vi "InitializeComms.vi"(4 "Inert MFC Channel":i32=8, 6 "Active MFC Channel":i32=7, 7 "Probe Target State":T1 {"Tset" format="%.1f"; "Telem" format="%.1f"; "GasC" format="%.1g"; "GasB" format="%.1f"; "GasA" format="%.1f"; "Z" format="%.3g"; "Y" format="%.3g"; "X" format="%.3g"; "RampRate" format="%.1f"}, 8 "error in":errorcluster, 9 "MFC channel":refnum<visa-resource-name>="COM2", 10 "Watlow channel":refnum<visa-resource-name>="COM3", 11 "Motor channel":refnum<visa-resource-name>="COM6") -> (0 "error out":errorcluster, 2 "Current probe state":T1 {"Tset" format="%.1f"; "Telem" format="%.1f"; "GasC" format="%.1g"; "GasB" format="%.1f"; "GasA" format="%.1f"; "Z" format="%.3g"; "Y" format="%.3g"; "X" format="%.3g"; "RampRate" format="%.1f"}, 3 "Probe Target State out":T1 {"Tset" format="%.1f"; "Telem" format="%.1f"; "GasC" format="%.1g"; "GasB" format="%.1f"; "GasA" format="%.1f"; "Z" format="%.3g"; "Y" format="%.3g"; "X" format="%.3g"; "RampRate" format="%.1f"})   [LabVIEW 2013]
uses:
  controls/Microprobe Vars.ctl
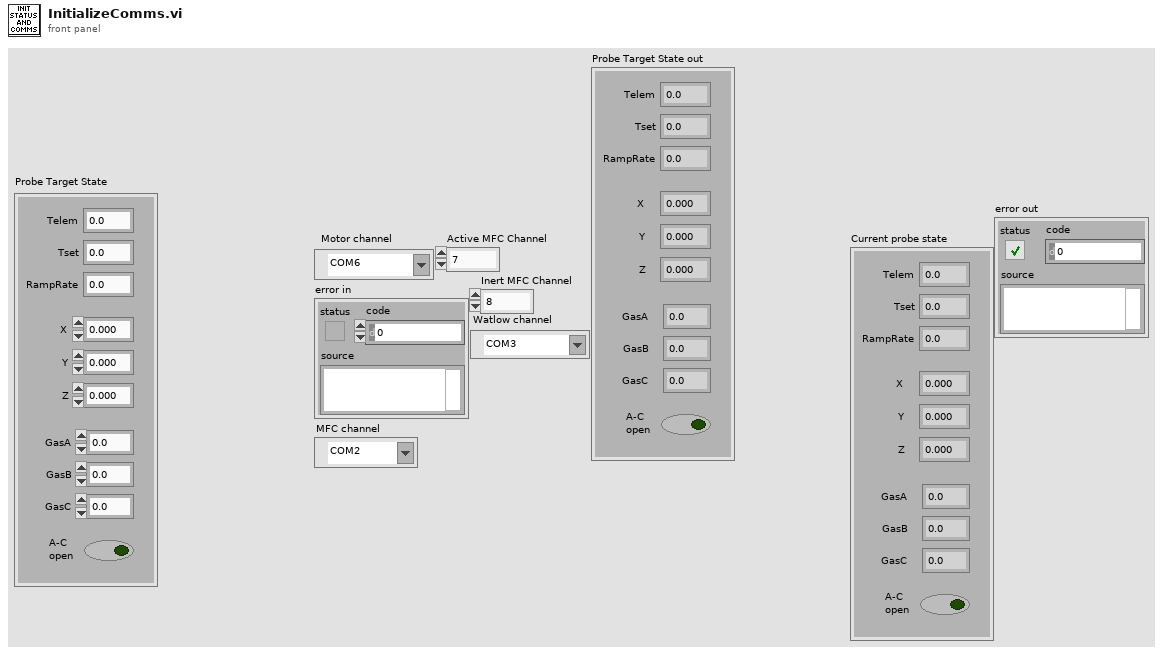
[diagram p1: front panel]
types:
  T1 = typedef "Microprobe Vars.ctl" = cluster{"Telem":dbl, "Tset":dbl, "RampRate":dbl, "X":dbl, "Y":dbl, "Z":dbl, "GasA":dbl, "GasB":dbl, "GasC":dbl, "A-C\nopen":bool}
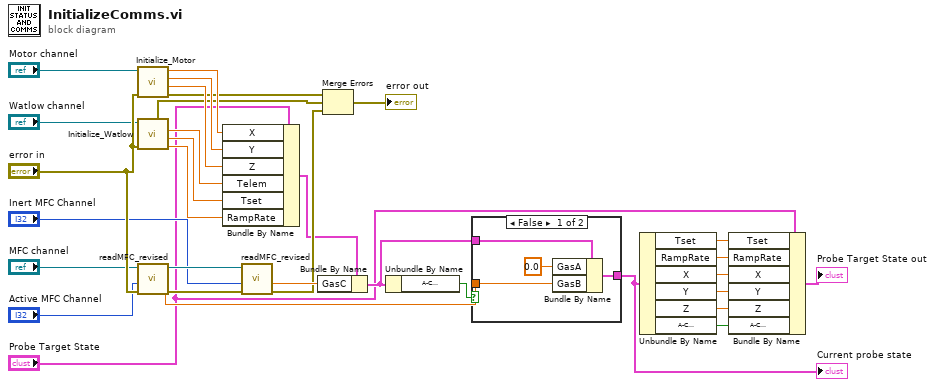
[diagram p0: block diagram]
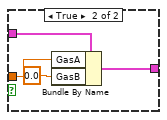
[diagram p2: hidden frame]
diagram:
  n1 = call <instrlib>:"Initialize_Motor.vi"("error in"="error in", "Motor channel"="Motor channel") -> ("error out"=w19:errorcluster, "Z"=w28:dbl, "Y"=w29:dbl, "X"=w30:dbl)  [unwired: 6 in]
  n2 = call <instrlib>:"Initialize_Watlow.vi"("Error In"="error in", "Watlow channel"="Watlow channel") -> ("Ramp rate"=w11:dbl, "Setpoint"=w12:dbl, "Current temp"=w13:dbl, "Error Out"=w18:errorcluster)  [unwired: 4 in, 1 out]
  n3 = call <instrlib>:"readMFC_revised.vi"("error in"="error in", "channel"="Active MFC Channel", "VISA resource name"="MFC channel") -> ("error out"=w31:errorcluster, "flow rate sccm"=w27:dbl, "VISA resource name out"=w32:refnum<visa-resource-name>)  [unwired: 6 in]
  n4 = Bundle By Name(cluster="Probe Target State", "X"=w30, "Y"=w29, "Z"=w28, "Telem"=w13, "Tset"=w12, "RampRate"=w11) -> (w10:T1)
  n5 = call <instrlib>:"readMFC_revised.vi"("error in"=w31, "channel"="Inert MFC Channel", "VISA resource name"=w32) -> ("error out"=w17:errorcluster, "flow rate sccm"=w25:dbl)  [unwired: 6 in, 1 out]
  n6 = Bundle By Name(cluster=w10, "GasC"=w25) -> (w24:T1)
  n7 = Merge Errors(w19, w18, w17) -> (→"error out":errorcluster)
  n8 = Unbundle By Name(w24) -> ("A-C\nopen"=w26:bool)
  n9 = case shown="False" w26 {
    tunnel: w27 -> [w36 w38]
    tunnel: w24 -> [w33 w40]
    tunnel: [w34 w39] -> w9
    frame False {
      n10 = Bundle By Name(cluster=w33, "GasA"=0.0, "GasB"=w36) -> (w34:T1)
    }
    frame True {
      n11 = Bundle By Name(cluster=w40, "GasA"=w38, "GasB"=0.0) -> (w39:T1)
    }
  }
  "Current probe state" <- w9
  n12 = Unbundle By Name(w9) -> ("Tset"=w8:dbl, "RampRate"=w7:dbl, "X"=w6:dbl, "Y"=w5:dbl, "Z"=w4:dbl, "A-C\nopen"=w1:bool)
  n13 = Bundle By Name(cluster="Probe Target State", "Tset"=w8, "RampRate"=w7, "X"=w6, "Y"=w5, "Z"=w4, "A-C\nopen"=w1) -> (→"Probe Target State out":T1)
